vi "principal.vi"() -> ()   [LabVIEW 2018]
uses:
  <vilib>/Instr/_visa.llb/Select Event Type.ctl
  <vilib>/Instr/_visa.llb/VISA Configure Serial Port (Instr).vi
  variablesglobales.vi
panel:
  out "Boolean":bool
  out "Numeric 2":dbl
  out "Waveform Graph":dbl[](graph)
  out "a":dbl
  out "Numeric":dbl
  out "String":string
  in  "stop":bool
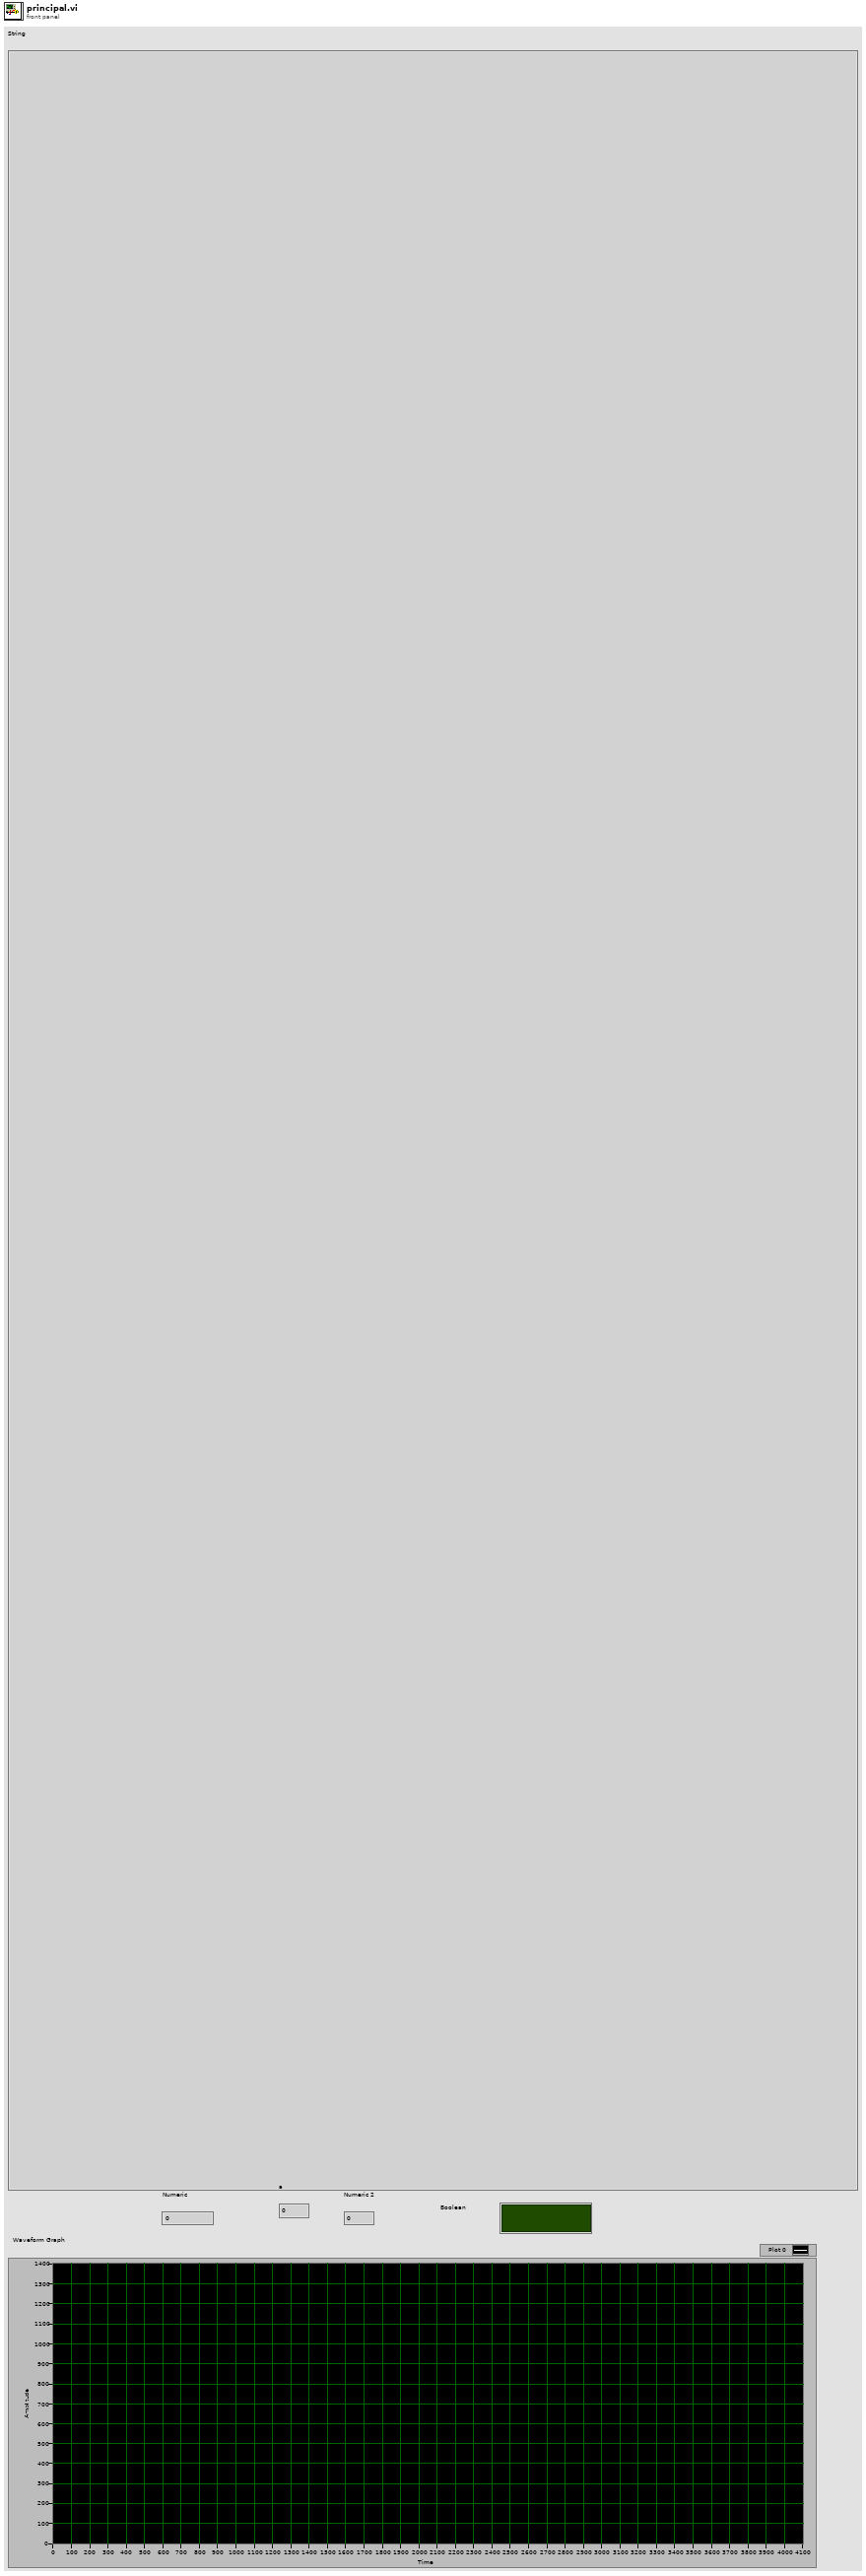
[diagram p1: front panel]
types:
  T1 = typedef "Select Event Type.ctl" = u32
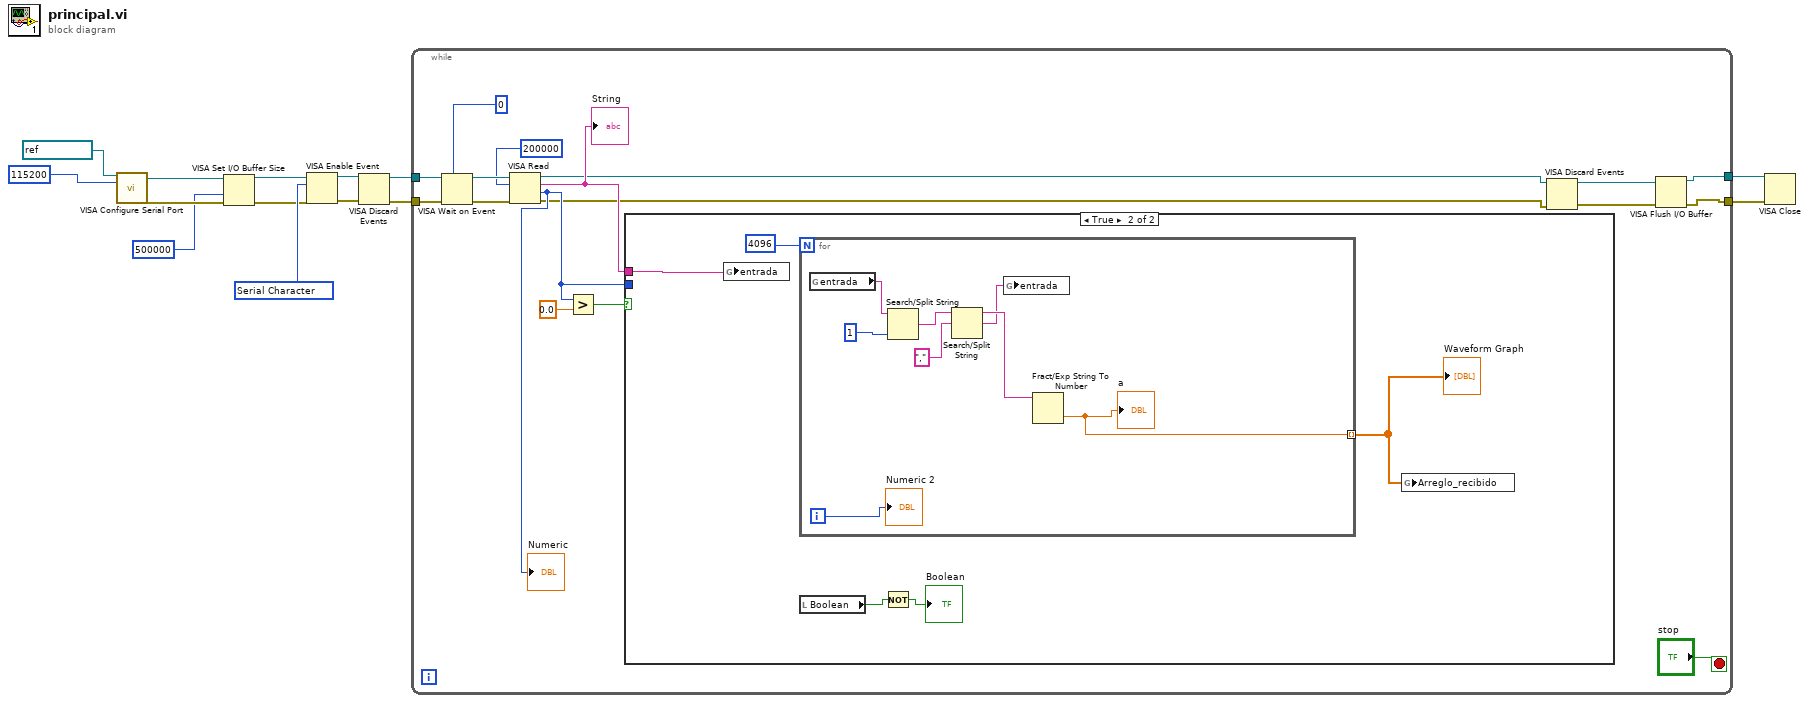
[diagram p0: block diagram]
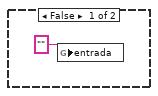
[diagram p2: hidden frame]
diagram:
  w8 = T1 1073684533 items=["Service Request"=1073684491, "Trigger"=3221168138, "Clear"=1073684493, "VXI Signal"=1073684512, "VXI/VME Interrupt"=3221168161, "VXI/VME Sysfail"=1073684509, "VXI/VME Sysreset"=1073684510, "GPIB CIC"=1073684498, "GPIB Talk"=1073684499, "GPIB Listen"=1073684500, "PXI Interrupt"=1073684514, "Serial Break"=1073684515, "Serial TermChar"=1073684516, "Serial CTS"=1073684521, "Serial DSR"=1073684522, "Serial DCD"=1073684524, "Serial RI"=1073684526, "Serial Character"=1073684533, "USB Interrupt"=1073684535, "All Enabled"=1073709055] ("Event Type")
  n1 = call-poly "VISA Configure Serial Port"("VISA resource name"=refnum<visa-resource-name> "COM20", "baud rate (9600)"=u32 115200) -> ("VISA resource name out"=w2:refnum<visa-resource-name>, "error out"=w3:errorcluster)  [unwired: 12 in]
  n2 = VISA Set I/O Buffer Size(VISA resource name=w2, size (4096)=u32 500000, error in (no error)=w3) -> (VISA resource name out=w5:refnum<visa-resource-name>, error out=w4:errorcluster)  [unwired: 1 in]
  n3 = VISA Enable Event(8:w4, 10:w8, 11:w5) -> (0:w12:errorcluster, 3:w11:refnum<visa-resource-name>)  [unwired: 1 in]
  n4 = VISA Discard Events(8:w12, 11:w11) -> (0:w10:errorcluster, 3:w9:refnum<visa-resource-name>)  [unwired: 2 in]
  n5 = while {
    tunnel: w10 -> [w31]
    tunnel: w9 -> [w30]
    tunnel: [w20] -> w7
    tunnel: [w19] -> w6
    stop <- "stop" stop-if-true
    n6 = VISA Wait on Event(7:u32 0 ("timeout (0)"), 8:w31, 11:w30) -> (0:w29:errorcluster, 3:w28:refnum<visa-resource-name>)  [unwired: 2 in, 2 out]
    n7 = VISA Read(VISA resource name=w28, byte count=u32 200000, error in (no error)=w29) -> (VISA resource name out=w15:refnum<visa-resource-name>, read buffer=w21:string, return count=w22:u32, error out=w16:errorcluster)
    "Numeric" <- w22
    "String" <- w21
    n8 = Greater?(x=w22, y=0.0) -> (0:w23:bool)
    n9 = case shown="True" w23 {
      tunnel: w21 -> [_ w33]
      tunnel: w22 -> [_ _]
      frame False {
        n10 = global write "variablesglobales.vi" "entrada"("" ("entrada")) -> ()
      }
      frame True {
        n11 = global write "variablesglobales.vi" "entrada"(w33) -> ()
        n12 = for {
          N: 4096 -> [_]
          tunnel: [w41] -> w36 mode=indexing
          i -> [w38]
          n13 = global read "variablesglobales.vi" "entrada"() -> (w39:string)
          n14 = Search/Split String(string=w39, offset (0)=1) -> (match + rest of string=w44:string)  [unwired: 1 in, 2 out]
          n15 = Search/Split String(string=w44, search string/char (-)=",") -> (substring before match=w42:string, match + rest of string=w40:string)  [unwired: 1 in, 1 out]
          n16 = global write "variablesglobales.vi" "entrada"(w40) -> ()
          n17 = Fract/Exp String To Number(string=w42) -> (number=w41:dbl)  [unwired: 3 in, 1 out]
          "a" <- w41
          "Numeric 2" <- w38
        }
        "Waveform Graph" <- w36
        n18 = local read "Boolean"() -> (w34:bool)
        n19 = Not(x=w34) -> (.not. x?=→"Boolean":bool)
        n20 = global write "variablesglobales.vi" "Arreglo_recibido"(w36) -> ()
      }
    }
    n21 = VISA Discard Events(8:w16, 11:w15) -> (0:w17:errorcluster, 3:w18:refnum<visa-resource-name>)  [unwired: 2 in]
    n22 = VISA Flush I/O Buffer(VISA resource name=w18, error in (no error)=w17) -> (VISA resource name out=w20:refnum<visa-resource-name>, error out=w19:errorcluster)  [unwired: 1 in]
  }
  n23 = VISA Close(VISA resource name=w7, error in (no error)=w6) -> ()  [unwired: 1 out]
